vi "字符串的ASCII码加减1.vi"(11 "原字符串":string) -> (2 "ASCII码":string)   [LabVIEW 2016, in "自动更新.lvlib" / "TCP文件传输系统.lvlib" / "TCP接收文件.lvlib"]
panel:
  out "数组":u8[](array[numeric])
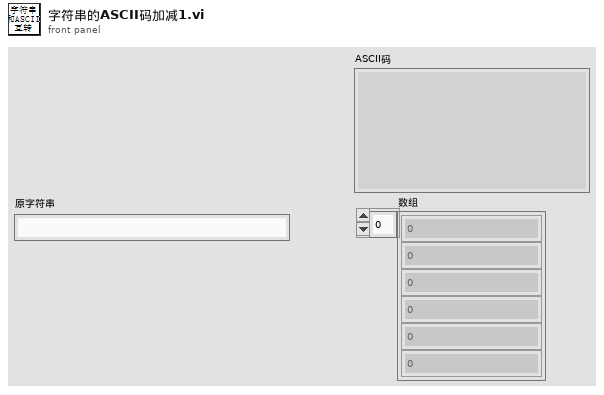
[diagram p1: front panel]
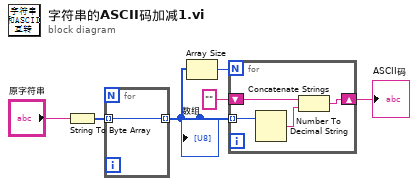
[diagram p0: block diagram]
diagram:
  n1 = String To Byte Array(string="原字符串") -> (unsigned byte array=w5:u8[])
  n2 = for {
    tunnel: w5 -> [w7] mode=indexing
    tunnel: [w7] -> w1 mode=indexing
  }
  "数组" <- w1
  n3 = Array Size(array=w1) -> (size(s)=w4:i32)
  n4 = for {
    N: w4 -> [_]
    shift-right: [w11] -> w3
    shift-left: "" -> [w10]
    tunnel: w1 -> [w9] mode=indexing
    n5 = Number To Decimal String(number=w9) -> (decimal integer string=w8:string)  [unwired: 1 in]
    n6 = Concatenate Strings(w10, w8) -> (w11:string)
  }
  "ASCII码" <- w3
